vi "QTMTest.vi"() -> ()   [LabVIEW 2010]
uses:
  CustomIO.ctl
panel:
  out "return count":u32
  in  "timeout ms (25000)":i32=6000
  out "Waveform Chart":dbl(graph)
  in  "SamplingRate [ms]":u32
  in  "stop":bool
  out "error out":errorcluster
  out "DataOut":dbl[](array[numeric])
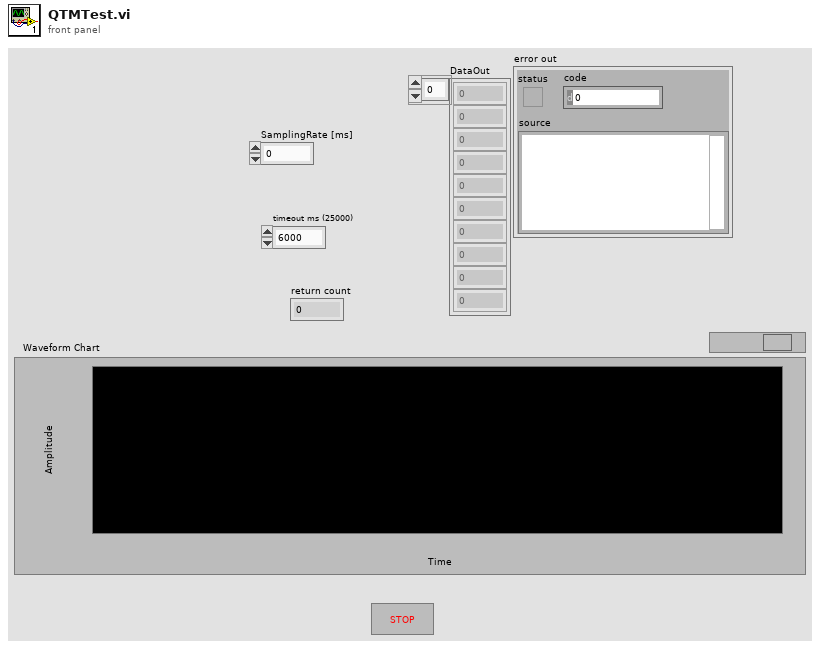
[diagram p1: front panel]
types:
  T1 = typedef "CustomIO.ctl" = enum16{"Init", "Read", "Write", "Close", "N/O"}
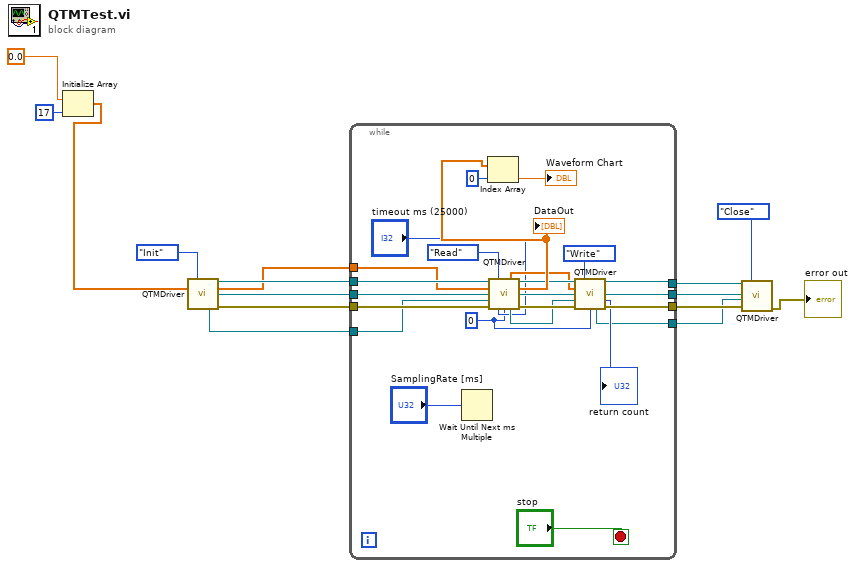
[diagram p0: block diagram]
diagram:
  n1 = Initialize Array(0.0, 17 ("dimension size")) -> (w2:dbl[])
  n2 = call "QTMDriver.vi"("Ring"=CustomIO."Init", "DataIn"=w2) -> ("connection ID out"=w14:refnum<k5>, "DataOut"=w1:dbl[], "QTMqueue Out"=w6:refnum<queue>, "VI Refnum QTMTask Out"=w5:refnum<vi>, "error out"=w13:errorcluster)  [unwired: 7 in, 2 out]
  n3 = while {
    tunnel: w14 -> [w38]
    tunnel: w13 -> [w37]
    tunnel: w1 -> [w36]
    tunnel: [w26] -> w9
    tunnel: [w28] -> w8
    tunnel: w6 -> [w21]
    tunnel: w5 -> [w20]
    tunnel: [w19] -> w4
    tunnel: [w18] -> w3
    stop <- "stop" stop-if-true
    w16 = 0 ("DataOutIndex")
    n4 = Wait Until Next ms Multiple(millisecond multiple="SamplingRate [ms]") -> ()  [unwired: 1 out]
    n5 = call "QTMDriver.vi"("connection ID"=w38, "Ring"=CustomIO."Read", "DataIn"=w36, "QTMqueue"=w21, "VI Refnum QTMTask"=w20, "error in"=w37, "timeout ms (25000)"="timeout ms (25000)", "DataOutIndex"=w16) -> ("ArrayOut"=w24:dbl[], "connection ID out"=w27:refnum<k5>, "DataOut"=w32:dbl[], "QTMqueue Out"=w23:refnum<queue>, "VI Refnum QTMTask Out"=w22:refnum<vi>, "error out"=w30:errorcluster)  [unwired: 1 in, 1 out]
    "DataOut" <- w32
    n6 = Index Array(array=w32, index=0) -> (element=→"Waveform Chart":dbl)
    n7 = call "QTMDriver.vi"("connection ID"=w27, "Ring"=CustomIO."Write", "DataIn"=w24, "QTMqueue"=w23, "VI Refnum QTMTask"=w22, "error in"=w30, "DataOutIndex"=w16) -> ("connection ID out"=w26:refnum<k5>, "QTMqueue Out"=w19:refnum<queue>, "return count"=→"return count":u32, "VI Refnum QTMTask Out"=w18:refnum<vi>, "error out"=w28:errorcluster)  [unwired: 2 in, 2 out]
  }
  n8 = call "QTMDriver.vi"("connection ID"=w9, "Ring"=CustomIO."Close", "QTMqueue"=w4, "VI Refnum QTMTask"=w3, "error in"=w8) -> ("error out"=→"error out":errorcluster)  [unwired: 4 in, 6 out]
